vi "WriteLog2File.vi"(8 "错误输入":errorcluster, 10 "文件路径（使用对话框）":path, 11 "文本":string) -> (0 "错误输出":errorcluster)   [LabVIEW 2018, in "RunningLog.lvclass"]
uses:
  RunningLog.lvclass
  <vilib>/Utility/error.llb/whitespace.ctl
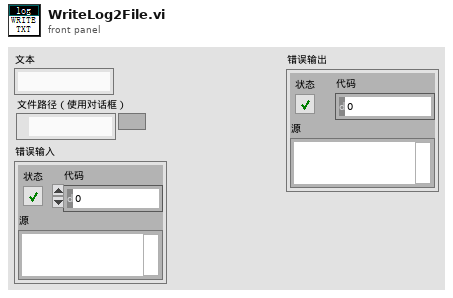
[diagram p1: front panel]
types:
  T1 = typedef "whitespace.ctl" = u16
  T2 = enum16{"open", "replace", "create", "open or create", "replace or create", "replace or create with confirmation"}
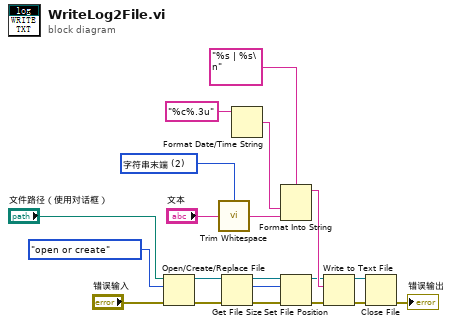
[diagram p0: block diagram]
diagram:
  w11 = T1 2 items=["两端", "字符串首端", "字符串末端"] ("location (both)")
  n1 = Open/Create/Replace File(file path (use dialog)="文件路径（使用对话框）", error in="错误输入", operation (0:open)=T2."open or create" ("操作(0:open)")) -> (refnum out=w7:refnum<file>, error out=w6:errorcluster)  [unwired: 3 in, 1 out]
  n2 = call <vilib>:"Trim Whitespace.vi"("string"="文本", "location (both)"=w11) -> ("trimmed string"=w9:string)
  n3 = Get File Size(file=w7, error in=w6) -> (refnum out=w5:refnum<file>, size (in bytes)=w1:i64, 0:w4:errorcluster)
  n4 = Format Date/Time String(time format string (%c)="%c%.3u" ("时间格式字符串(%c)")) -> (date/time string=w10:string)  [unwired: 2 in]
  n5 = Format Into String(format string="%s | %s\n" ("格式字符串"), w10, w9) -> (resulting string=w8:string)  [unwired: 2 in, 1 out]
  n6 = Set File Position(offset (in bytes) (0)=w1, refnum=w5, error in=w4) -> (refnum out=w2:refnum<file>, error out=w3:errorcluster)  [unwired: 1 in]
  n7 = Write to Text File(file (use dialog)=w2, text=w8, error in=w3) -> (refnum out=w19:refnum<file>, error out=w20:errorcluster)  [unwired: 1 in, 1 out]
  n8 = Close File(refnum=w19, error in=w20) -> (error out=→"错误输出":errorcluster)  [unwired: 1 out]
